vi "Read.vi"(8 "error in (no error)":errorcluster, 11 "Set Var Command Config in":refnum<class "Set Var Command Config.lvclass">) -> (0 "error out":errorcluster, 1 "Value":dbl, 2 "Var":string, 3 "Set Var Command Config out":refnum<class "Set Var Command Config.lvclass">)   [LabVIEW 2020, in "VolatusSeqConfig.lvlib" / "Set Var Command Config.lvclass"]
uses:
  Set Var Command Config.lvclass
  Set Var Command Config.lvclass/Set Var Command Config.ctl
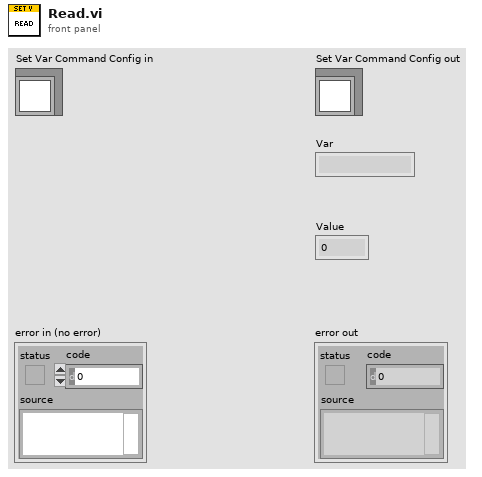
[diagram p1: front panel]
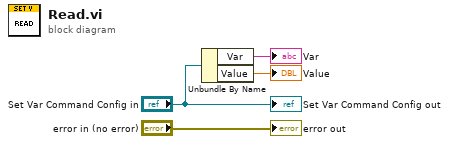
[diagram p0: block diagram]
diagram:
  n1 = Unbundle By Name("Set Var Command Config in") -> ("Var"=→"Var":string, "Value"=→"Value":dbl)
  "error out" <- "error in (no error)"
  "Set Var Command Config out" <- "Set Var Command Config in"
